vi "Interpolate by Distance.vi"() -> ()   [LabVIEW 2019]
panel:
  in  "Distance":dbl
  in  "Points":cluster{"X":dbl, "Y":dbl}[](array[cluster])
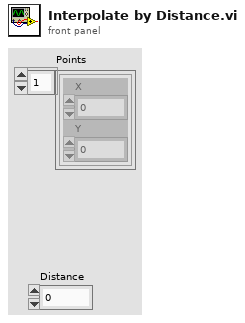
[diagram p1: front panel]
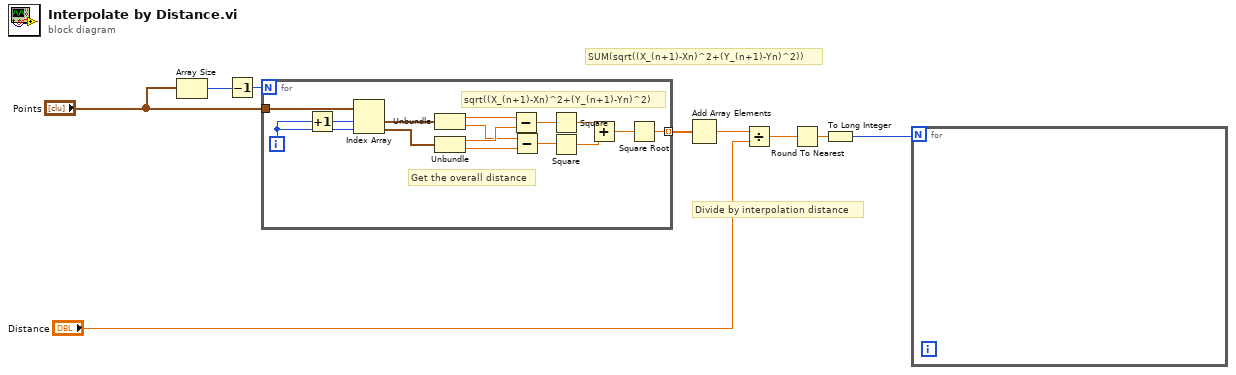
[diagram p0: block diagram]
diagram:
  # "SUM(sqrt((X_(n+1)-Xn)^2+(Y_(n+1)-Yn)^2))"
  # "Divide by interpolation distance"
  n1 = Array Size(array="Points") -> (size(s)=w8:i32)
  n2 = Decrement(x=w8) -> (x-1=w7:i32)
  n3 = for {
    N: w7 -> [_]
    tunnel: "Points" -> [w24]
    tunnel: [w10] -> w6 mode=indexing
    i -> [w22]
    # "sqrt((X_(n+1)-Xn)^2+(Y_(n+1)-Yn)^2)"
    # "Get the overall distance"
    n4 = Increment(x=w22) -> (x+1=w23:i32)
    n5 = Index Array(array=w24, index #1=w23, index #2=w22) -> (element #1=w21:cluster{"X":dbl, "Y":dbl}, element #2=w20:cluster{"X":dbl, "Y":dbl})
    n6 = Unbundle(w21) -> ("X"=w19:dbl, "Y"=w17:dbl)
    n7 = Unbundle(w20) -> ("X"=w18:dbl, "Y"=w16:dbl)
    n8 = Subtract(x=w19, y=w18) -> (x-y=w15:dbl)
    n9 = Subtract(x=w17, y=w16) -> (x-y=w14:dbl)
    n10 = Square(x=w15) -> (x^2=w13:dbl)
    n11 = Square(x=w14) -> (x^2=w12:dbl)
    n12 = Add(x=w13, y=w12) -> (x+y=w11:dbl)
    n13 = Square Root(x=w11) -> (sqrt(x)=w10:dbl)
  }
  n14 = Add Array Elements(numeric array=w6) -> (sum=w5:dbl)
  n15 = Divide(x=w5, y="Distance") -> (x/y=w3:dbl)
  n16 = Round To Nearest(number=w3) -> (nearest integer value=w2:dbl)
  n17 = To Long Integer(number=w2) -> (32bit integer=w1:i32)
  n18 = for {
    N: w1 -> [_]
  }
